vi "test_libssh2_session_banner_set.vi"() -> ()   [LabVIEW 2013, in "libssh2_integration_tests.lvlib"]
uses:
  libssh2_integration_tests.lvlib
  libssh2/libssh2_init_default.vi
  libssh2/libssh2_session_handshake_tcp.vi
  libssh2/libssh2.lvlib
  <vilib>/addons/_JKI Toolkits/Caraya/classes/Test/Test.lvclass
  <vilib>/addons/_JKI Toolkits/Caraya/classes/Assert/Assert.lvclass
panel:
  out "error out":errorcluster
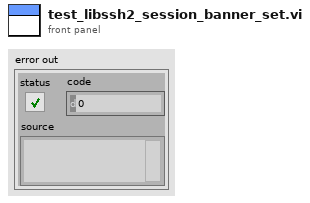
[diagram p1: front panel]
types:
  T1 = typedef "libssh2.lvlib/Session Refnum.ctl" = refnum<k1>
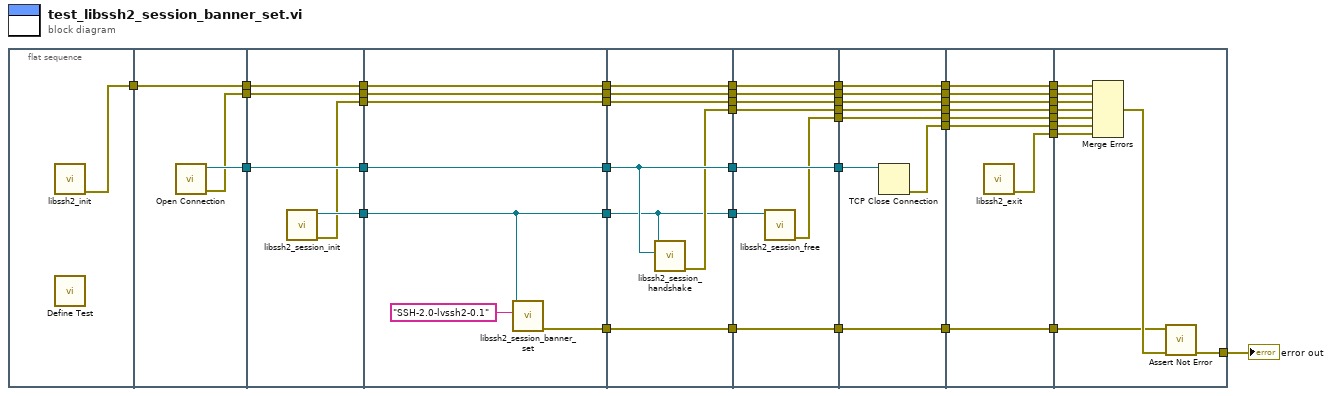
[diagram p0: block diagram]
diagram:
  n1 = flat-sequence {
    tunnel: [w46] -> w45
    tunnel: [w49] -> w44
    tunnel: w45 -> [w48]
    tunnel: [w48] -> w43
    tunnel: [w47] -> w42
    tunnel: w44 -> [w54]
    tunnel: [w54] -> w30
    tunnel: w43 -> [w53]
    tunnel: [w53] -> w28
    tunnel: w42 -> [w52]
    tunnel: [w52] -> w26
    tunnel: [w51] -> w24
    tunnel: [w50] -> w22
    tunnel: w30 -> [w61]
    tunnel: [w61] -> w29
    tunnel: w28 -> [w60]
    tunnel: [w60] -> w27
    tunnel: w26 -> [w59]
    tunnel: [w59] -> w25
    tunnel: w24 -> [w57]
    tunnel: [w57] -> w23
    tunnel: w22 -> [w58]
    tunnel: [w58] -> w21
    tunnel: [w55] -> w11
    tunnel: w29 -> [w65]
    tunnel: [w65] -> w7
    tunnel: w27 -> [w68]
    tunnel: [w68] -> w6
    tunnel: w25 -> [w67]
    tunnel: [w67] -> w5
    tunnel: w23 -> [w62]
    tunnel: w21 -> [w66]
    tunnel: [w66] -> w4
    tunnel: [w64] -> w3
    tunnel: w11 -> [w63]
    tunnel: [w63] -> w2
    tunnel: [w62] -> w1
    tunnel: w7 -> [w76]
    tunnel: [w76] -> w20
    tunnel: w6 -> [w75]
    tunnel: [w75] -> w19
    tunnel: w5 -> [w74]
    tunnel: [w74] -> w18
    tunnel: w4 -> [w73]
    tunnel: [w73] -> w17
    tunnel: w3 -> [w72]
    tunnel: [w72] -> w16
    tunnel: [w71] -> w13
    tunnel: w2 -> [w70]
    tunnel: [w70] -> w10
    tunnel: w1 -> [w69]
    tunnel: w20 -> [w84]
    tunnel: w19 -> [w83]
    tunnel: [w83] -> w41
    tunnel: w18 -> [w82]
    tunnel: [w82] -> w40
    tunnel: [w81] -> w39
    tunnel: w17 -> [w80]
    tunnel: [w80] -> w38
    tunnel: w16 -> [w79]
    tunnel: [w79] -> w37
    tunnel: [w78] -> w14
    tunnel: w13 -> [w78]
    tunnel: w10 -> [w77]
    tunnel: [w77] -> w9
    tunnel: w41 -> [w92]
    tunnel: [w92] -> w36
    tunnel: w40 -> [w91]
    tunnel: [w91] -> w35
    tunnel: w39 -> [w90]
    tunnel: [w90] -> w34
    tunnel: [w89] -> w33
    tunnel: w38 -> [w88]
    tunnel: [w88] -> w32
    tunnel: w37 -> [w87]
    tunnel: [w87] -> w31
    tunnel: [w86] -> w15
    tunnel: w14 -> [w86]
    tunnel: w9 -> [w85]
    tunnel: [w85] -> w8
    tunnel: w36 -> [w102]
    tunnel: w35 -> [w101]
    tunnel: w34 -> [w100]
    tunnel: w33 -> [w99]
    tunnel: w32 -> [w98]
    tunnel: [w96] -> w12
    tunnel: w31 -> [w95]
    tunnel: w15 -> [w94]
    tunnel: w8 -> [w93]
    frame #0 {
      n2 = call-poly "libssh2_init.vi"() -> ("error out"=w46:errorcluster)  [unwired: 11 in]
      n3 = call <vilib>:"Define Test.vi"() -> ()  [unwired: 10 in, 2 out]
    }
    frame #1 {
      n4 = call "Open Connection.vi"() -> ("error out"=w47:errorcluster, "connection ID"=w49:refnum<k5>)  [unwired: 10 in]
    }
    frame #2 {
      n5 = call "libssh2_session_init.vi"() -> ("error out"=w50:errorcluster, "session"=w51:T1)  [unwired: 10 in]
    }
    frame #3 {
      n6 = call "libssh2_session_banner_set.vi"("banner"="SSH-2.0-lvssh2-0.1", "session"=w57) -> ("error out"=w55:errorcluster)  [unwired: 9 in]
    }
    frame #4 {
      n7 = call-poly "libssh2_session_handshake.vi"("tcp connection"=w65, "session"=w62) -> ("error out"=w64:errorcluster)  [unwired: 9 in]
    }
    frame #5 {
      n8 = call "libssh2_session_free.vi"("session"=w69) -> ("error out"=w71:errorcluster)  [unwired: 10 in]
    }
    frame #6 {
      n9 = TCP Close Connection(connection ID=w84) -> (error out=w81:errorcluster)  [unwired: 2 in, 1 out]
    }
    frame #7 {
      n10 = call "libssh2_exit.vi"() -> ("error out"=w89:errorcluster)  [unwired: 11 in]
    }
    frame #8 {
      n11 = Merge Errors(w102, w101, w98, w95, w94, w100, w99) -> (w97:errorcluster)
      n12 = call <vilib>:"Assert Not Error.vi"("error in (no error)"=w97, "Not Error?"=w93) -> ("error out"=w96:errorcluster)  [unwired: 8 in, 1 out]
    }
  }
  "error out" <- w12
